vi "Linear Temperature Image_v1.vi"() -> ()   [LabVIEW 2015]
doc: "An example of how you can get different types of images from the camera.\n\nNOTE: You must have ThermoVision installed to run this example."
uses:
  <userlib>/ThermoVision/ThermoVision.llb/Thermovision CameraTypes.ctl
  <userlib>/ThermoVision/ThermoVision.llb/ThermoVision DeviceTypes.ctl
  <userlib>/ThermoVision/ThermoVision.llb/ThermoVision CommunicationInterfaceType.ctl
  <userlib>/ThermoVision/ThermoVision Digital.llb/ThermoVision Digital ImageMode.ctl
  <userlib>/ThermoVision/ThermoVision Digital.llb/ThermoVision Digital ImageType.ctl
  <vilib>/Analysis/Matrix/Numeric/Conversions/Matrix To Array - RM.vi
  <vilib>/Analysis/Matrix/NI_Matrix.lvlib
panel:
  out "Camera":T1(plugin-control)
  in  "Kelvin Multiplier":dbl=10.0
  out "Celsius":dbl
  in  "Height":dbl=80.0
  in  "Width":dbl=80.0
  in  "Measure Box Y":dbl
  in  "Measure Box X":dbl
  out "Average":dbl
  out "Total":dbl
  out "Image(U16)":u16[][](array[numeric])
  in  "Image Mode":T2=enum."Temperature (0.1K)"
  in  "Interface":T3=enum."UVC"
  in  "Device":T4=enum."USB video"
  in  "Camera Serial Number":string
  in  "CameraType":T5=enum."FLIR A615/A645/SC645/SC655"
  in  "error in (no error)":errorcluster
  in  "Stop":bool
  out "error out":errorcluster
  # "Note:\n Before running this VI\n 1. Select camera type supporting \n      linear temperature image (A-series)\n 2. Type camera serial number, if you \n     have more than one firewire camera\n     connected.\n 3. Run the VI\n 4. Press Stop button to terminate \n     VI-execution"
  # "Pre-run settings"
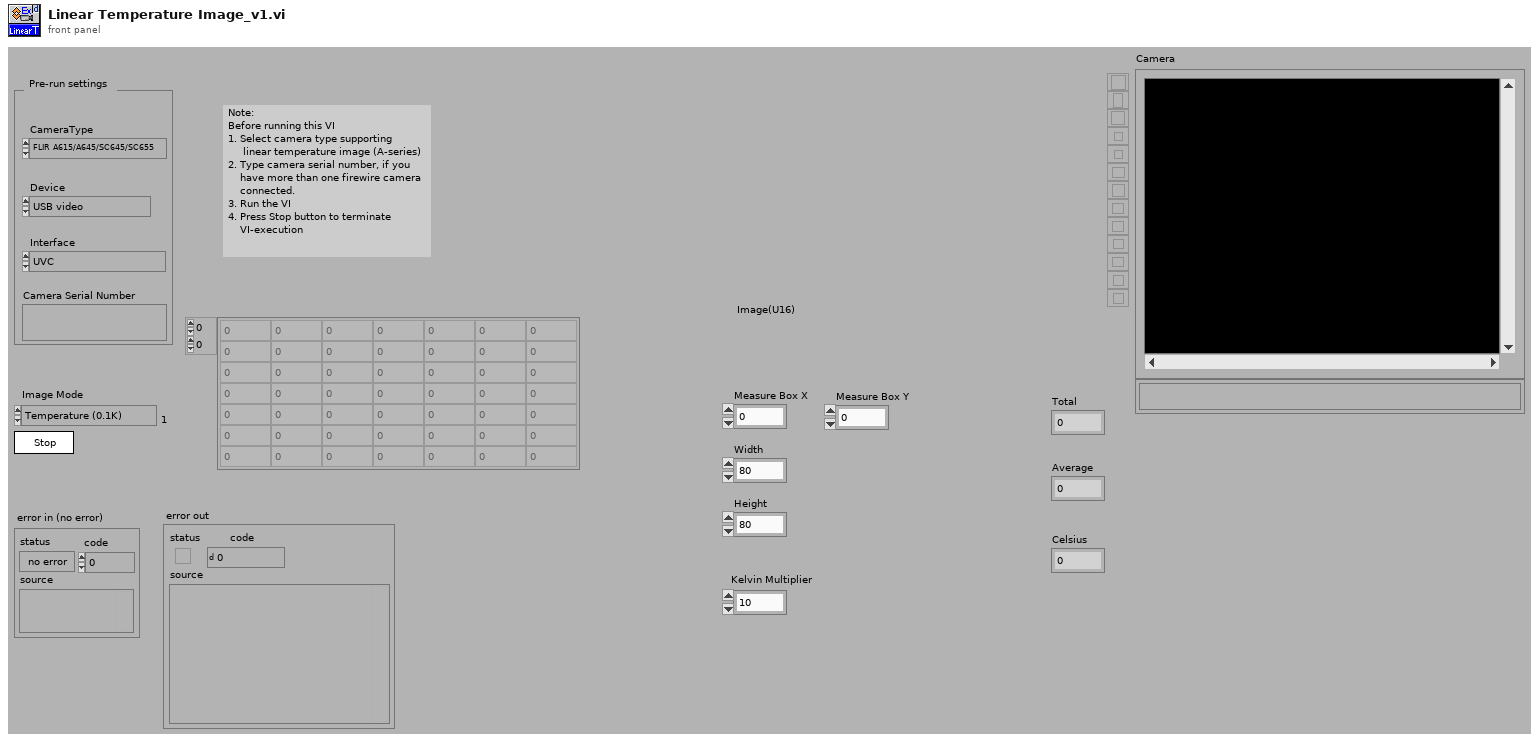
[diagram p1: front panel]
types:
  T1 = typedef "IMAQ Image.ctl" = refnum<image>
  T2 = typedef "ThermoVision Digital ImageMode.ctl" = enum16{"Signal", "Temperature (0.1K)", "Temperature (0.01K)"}
  T3 = typedef "ThermoVision CommunicationInterfaceType.ctl" = enum16{"File Only", "RS232", "TCP/IP(Ethernet)", "AV/C(FireWire)", "Gigabit Ethernet", "AXIS Video Server(Ethernet)", "UVC"}
  T4 = typedef "ThermoVision DeviceTypes.ctl" = enum16{"No Device", "FLIR PCCard", "ITEX IC-DIG 16", "Firewire 16-bit images", "Firewire 8-bit images", "Ethernet 16-bit images", "Ethernet 8-bit images", "IR-FlashLink", "iPort/GEV", "USB video"}
  T5 = typedef "Thermovision CameraTypes.ctl" = enum16{"ThermaCAM SC2000/SC3000", "THV 320/160", "ThermaCAM SC1000", "ThermaCAM S40/S45/S60/S65", "Thermovision A20/A40", "Cumulus SC4000/SC6000", "ThermaCAM SC640/SC660", "FLIR A320/A300/A310", "FLIR A325(A320G)/A315/SC305/SC325", "Indigo Merlin", "Indigo Phoenix", "Indigo Omega", "THV 1000", "THV 900", "FLIR GF320/GF309", "FLIR T-series", "FLIR A615/A645/SC645/SC655", "FLIR Exx series", "FLIR T620/T640/T420/T440"}
  T6 = enum16{"Internal Image Correction", "External Image Correction", "Auto Adjust", "Show Camera Info Dialog", "Show Device Status Dialog", "Reload Calibration(SC1000 only)"}
  T7 = enum16{"Unused0", "Unused1", "Unused2", "Unused3", "Unused4", "Unused5", "Unused6", "U16 Grayscale"}
  T8 = typedef "ThermoVision Digital ImageType.ctl" = enum16{"Raw", "Absolute", "Object", "Temperature", "Raw 8 bits"}
  T9 = typedef "Thermovision Object Reference.ctl" = refnum<k1>
  T10 = cluster{"Measure Box X":dbl, "Measure Box Y":dbl, dbl, dbl}
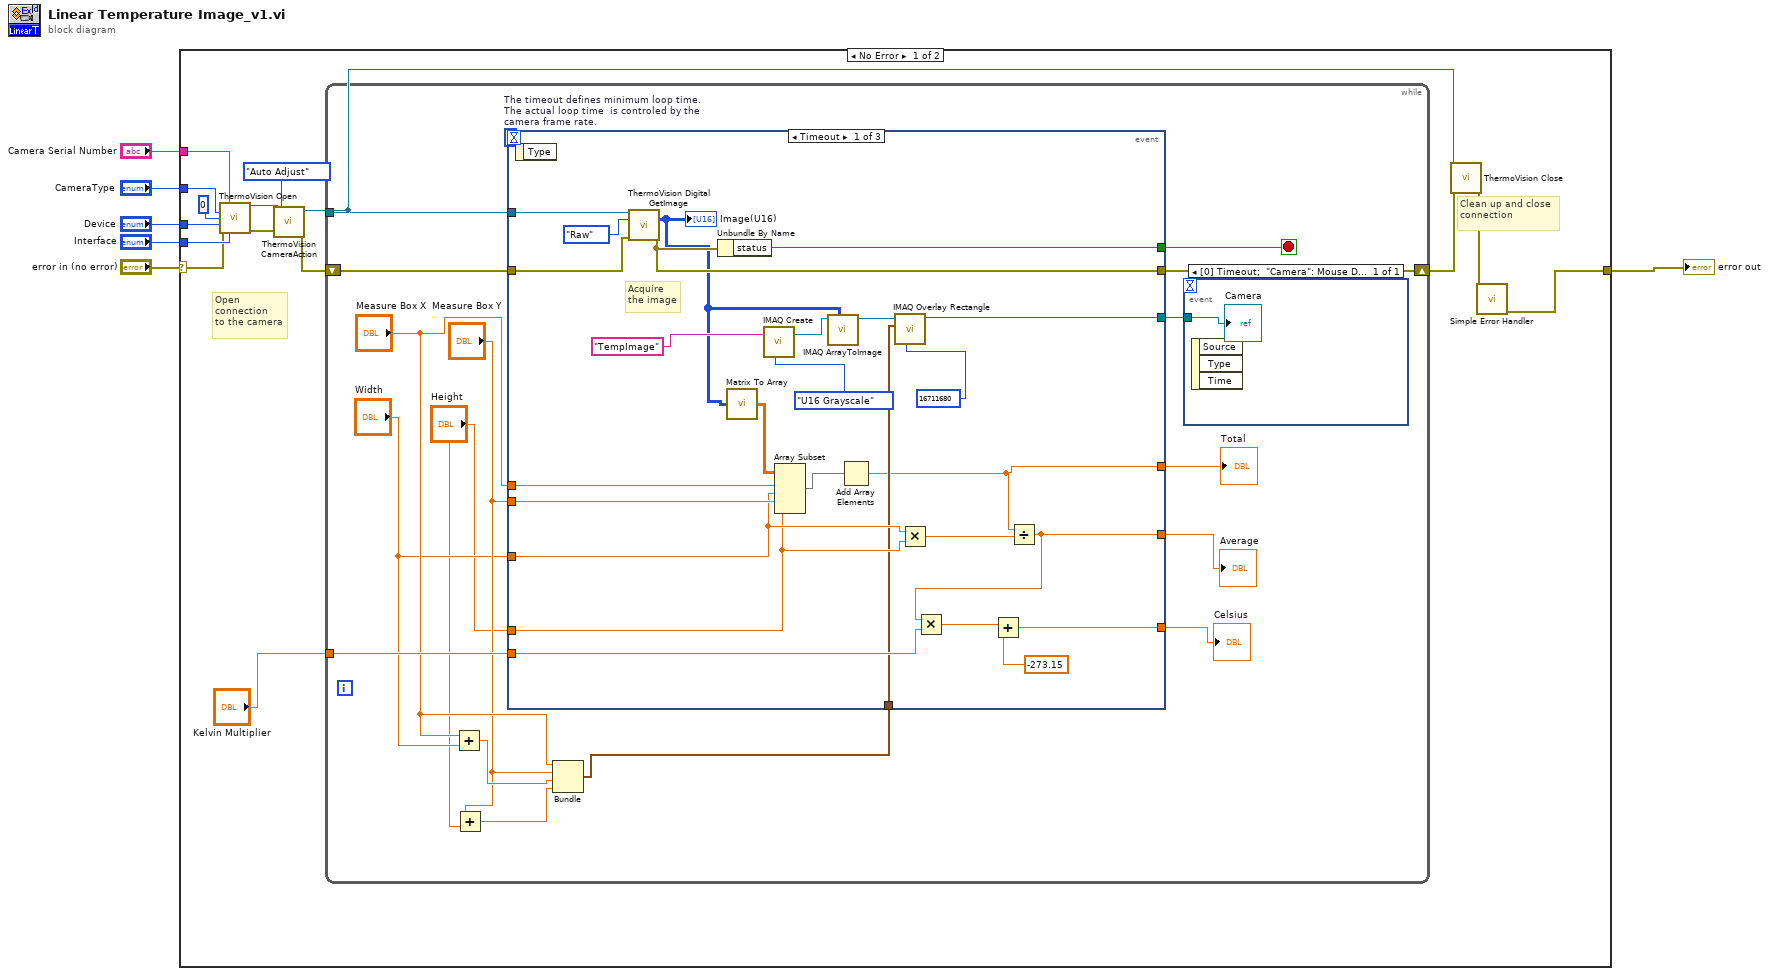
[diagram p0: block diagram]
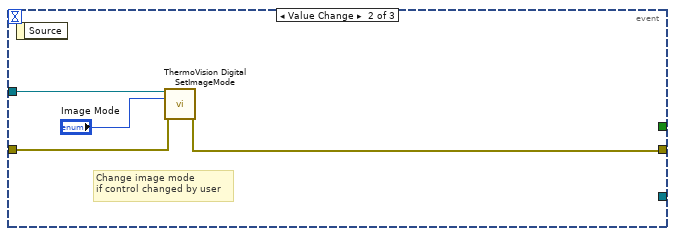
[diagram p2: hidden frame]
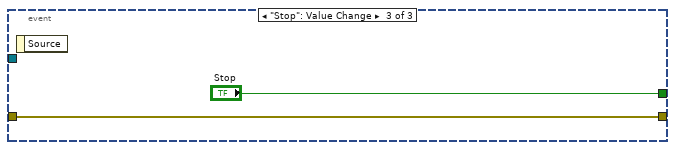
[diagram p3: hidden frame]
diagram:
  n1 = case shown="No Error" "error in (no error)" {
    selector: "error in (no error)" -> [w8 w72]
    tunnel: "CameraType" -> [w21 _]
    tunnel: [w19 w72] -> w5
    tunnel: "Camera Serial Number" -> [w17 _]
    tunnel: "Device" -> [w16 _]
    tunnel: "Interface" -> [w15 _]
    frame No Error {
      # "Open \nconnection\nto the camera"
      # "Clean up and close\nconnection"
      n2 = call <userlib>:"ThermoVision Open.vi"("Server/SN"=w17, "CameraType"=w21, "Port"=i16 0, "Device"=w16, "error in (no error)"=w8, "Interface"=w15) -> ("reference"=w14:T9, "error out"=w12:errorcluster)  [unwired: 8 in]
      n3 = call <userlib>:"ThermoVision CameraAction.vi"("error in (no error)"=w12, "Action"=T6."Auto Adjust", "reference"=w14) -> ("error out"=w10:errorcluster, "duplicate reference"=w13:T9)  [unwired: 7 in]
      n4 = while {
        shift-right: [w37] -> w9
        shift-left: w10 -> [w36]
        tunnel: w13 -> [w38]
        tunnel: "Kelvin Multiplier" -> [w33]
        stop <- w34 stop-if-true
        w35 = 5  # The timeout defines minimum loop time.  The actual loop time  is controled by the camera frame rate.
        n5 = Add(x="Measure Box X", y="Width") -> (x+y=w30:dbl)
        n6 = Add(x="Measure Box Y", y="Height") -> (x+y=w32:dbl)
        n7 = Bundle("Measure Box X"="Measure Box X", "Measure Box Y"="Measure Box Y", w30, w32) -> (w31:T10)  [unwired: 1 in]
        n8 = event shown="[0] Timeout" {
          selector: _ -> [_ _ _]
          dyn-events: _ -> [_ _ _]
          timeout: w35 -> [_ _ _]
          tunnel: w36 -> [w61 w69 w70]
          tunnel: w38 -> [w64 w68 _]
          tunnel: [w63 w67 w70] -> w37
          tunnel: [w62 _ "Stop"] -> w34
          tunnel: "Measure Box X" -> [w56 _ _]
          tunnel: "Measure Box Y" -> [w55 _ _]
          tunnel: "Width" -> [w53 _ _]
          tunnel: "Height" -> [w52 _ _]
          tunnel: w33 -> [w54 _ _]
          tunnel: w31 -> [w50 _ _]
          tunnel: [w43 _ _] -> w29
          tunnel: [w42 _ _] -> w28
          tunnel: [w41 _ _] -> w27
          tunnel: [w40 _ _] -> w22
          event Timeout {
            # "Acquire\nthe image"
            n9 = event-data() -> ()  [unwired: 1 in, 1 out]
            n10 = call <userlib>:"ThermoVision Digital GetImage.vi"("reference"=w64, "ImageType"=ThermoVision_Digital_ImageType."Raw", "error in (no error)"=w61) -> ("Image(U16)"=w45:u16[][], "error out"=w63:errorcluster)  [unwired: 7 in, 4 out]
            "Image(U16)" <- w45
            n11 = Unbundle By Name(w63) -> ("status"=w62:bool)
            n12 = call-poly <vilib>:"Matrix To Array.vi"("Real Matrix"=w45) -> ("Real 2D Array"=w51:dbl[][])
            n13 = call "IMAQ Create"("Image Name"="TempImage", "Image Type"=T7."U16 Grayscale") -> ("New Image"=w48:T1)  [unwired: 3 in, 1 out]
            n14 = Array Subset(array=w51, index (row)=w56, length (row)=w53, index (col)=w55, length (col)=w52) -> (w60:dbl[][])
            n15 = call "IMAQ ArrayToImage"("Image Pixels (U16)"=w45, "Image"=w48) -> ("Image Out"=w49:T1)  [unwired: 8 in, 1 out]
            n16 = Add Array Elements(numeric array=w60) -> (sum=w42:dbl)
            n17 = call "IMAQ Overlay Rectangle"("Color"=16711680, "Rectangle"=w50, "Image"=w49) -> ("Image Out"=w40:T1)  [unwired: 7 in, 1 out]
            n18 = Multiply(x=w53, y=w52) -> (x*y=w59:dbl)
            n19 = Divide(x=w42, y=w59) -> (x/y=w41:dbl)
            n20 = Multiply(x=w41, y=w54) -> (x*y=w58:dbl)
            n21 = Add(x=w58, y=-273.15) -> (x+y=w43:dbl)
          }
          event Value Change {
            # "Change image mode\nif control changed by user"
            n22 = event-data() -> ()  [unwired: 1 in, 1 out]
            n23 = call <userlib>:"ThermoVision Digital SetImageMode.vi"("reference"=w68, "Image Mode"="Image Mode", "error in (no error)"=w69) -> ("error out"=w67:errorcluster)  [unwired: 11 in, 1 out]
          }
          event "Stop": Value Change {
            n24 = event-data() -> ()  [unwired: 1 in, 1 out]
          }
        }
        "Total" <- w28
        "Average" <- w27
        "Celsius" <- w29
        n25 = event shown="[0] Timeout;  \"Camera\": Mouse Down" {
          selector: _ -> [_]
          dyn-events: _ -> [_]
          timeout: _ -> [_]
          tunnel: w22 -> [w39]
          event Timeout; "Camera": Mouse Down {
            n26 = event-data() -> ()  [unwired: 1 in, 3 out]
            "Camera" <- w39
          }
        }
      }
      n27 = call <userlib>:"ThermoVision Close.vi"("reference"=w13, "error in (no error)"=w9) -> ("error out"=w20:errorcluster)  [unwired: 13 in]
      n28 = call <vilib>:"Simple Error Handler.vi"("error in (no error)"=w20) -> ("error out"=w19:errorcluster)  [unwired: 4 in, 4 out]
    }
    frame Error {
    }
  }
  "error out" <- w5
